vi "GraphForm (SubVI).vi"(0 "R":T1, 2 "T":T1, 5 "error in":errorcluster, 10 "Title":string) -> (19 "error out":errorcluster)   [LabVIEW 2013]
panel:
  in  "1_ch_visible":bool=TRUE
  in  "2_ch_visible":bool=TRUE
  in  "3_ch_visible":bool=TRUE
  in  "4_ch_visible":bool=TRUE
  in  "5_ch_visible":bool=TRUE
  in  "6_ch_visible":bool=TRUE
  in  "7_ch_visible":bool=TRUE
  in  "8_ch_visible":bool=TRUE
  in  "Tab Control":enum32{"Page 2"}(tab)
  in  "Autoscale":bool=TRUE
  in  "Т max":u16=300 min=2 max=500 step=1
  in  "Т min":u16=3 min=1 max=350
  in  "R max":u16=6000 min=2 max=10000 step=1
  in  "R min":u16=100 min=1 max=350
  out "часы":string="0"
  in  "Добавить время":dbl(ring)=300.0 items=["1 мин."=60.0, "5 мин."=300.0, "20 мин."=1200.0]
  out "мин.":string="1"
  in  "xScale +":bool
  in  "xScale -":bool
  out "Graphs T":dynamicdata(graph)
  out "Graphs R":dynamicdata(graph)
  # "Шкала Т"
  # "Шкала R"
  # "Интервал просмотра"
  # ":"
  # "Канал"
  # "R [Ом]"
  # "Температура, К"
  # "Сопротивление, Ом"
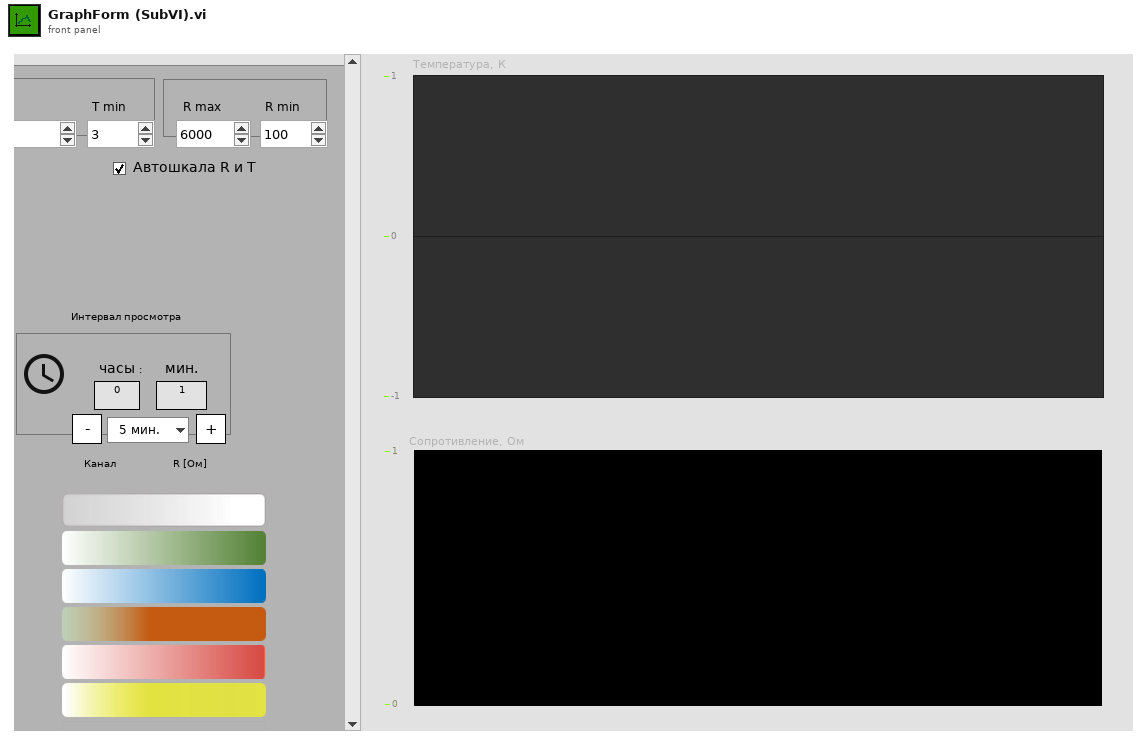
[diagram p1: front panel]
types:
  T1 = cluster{" R1":dbl, " R2":dbl, " R3":dbl, " R4":dbl, " R5":dbl, "R6":dbl, " R7":dbl, "R8":dbl}
  T2 = typedef "LVDateTimeRec.ctl" = cluster{"fractional second":dbl, "second":i32, "minute":i32, "hour":i32, "day of month":i32, "month":i32, "year":i32, "day of week":i32, "day of year":i32, "DST":i32}
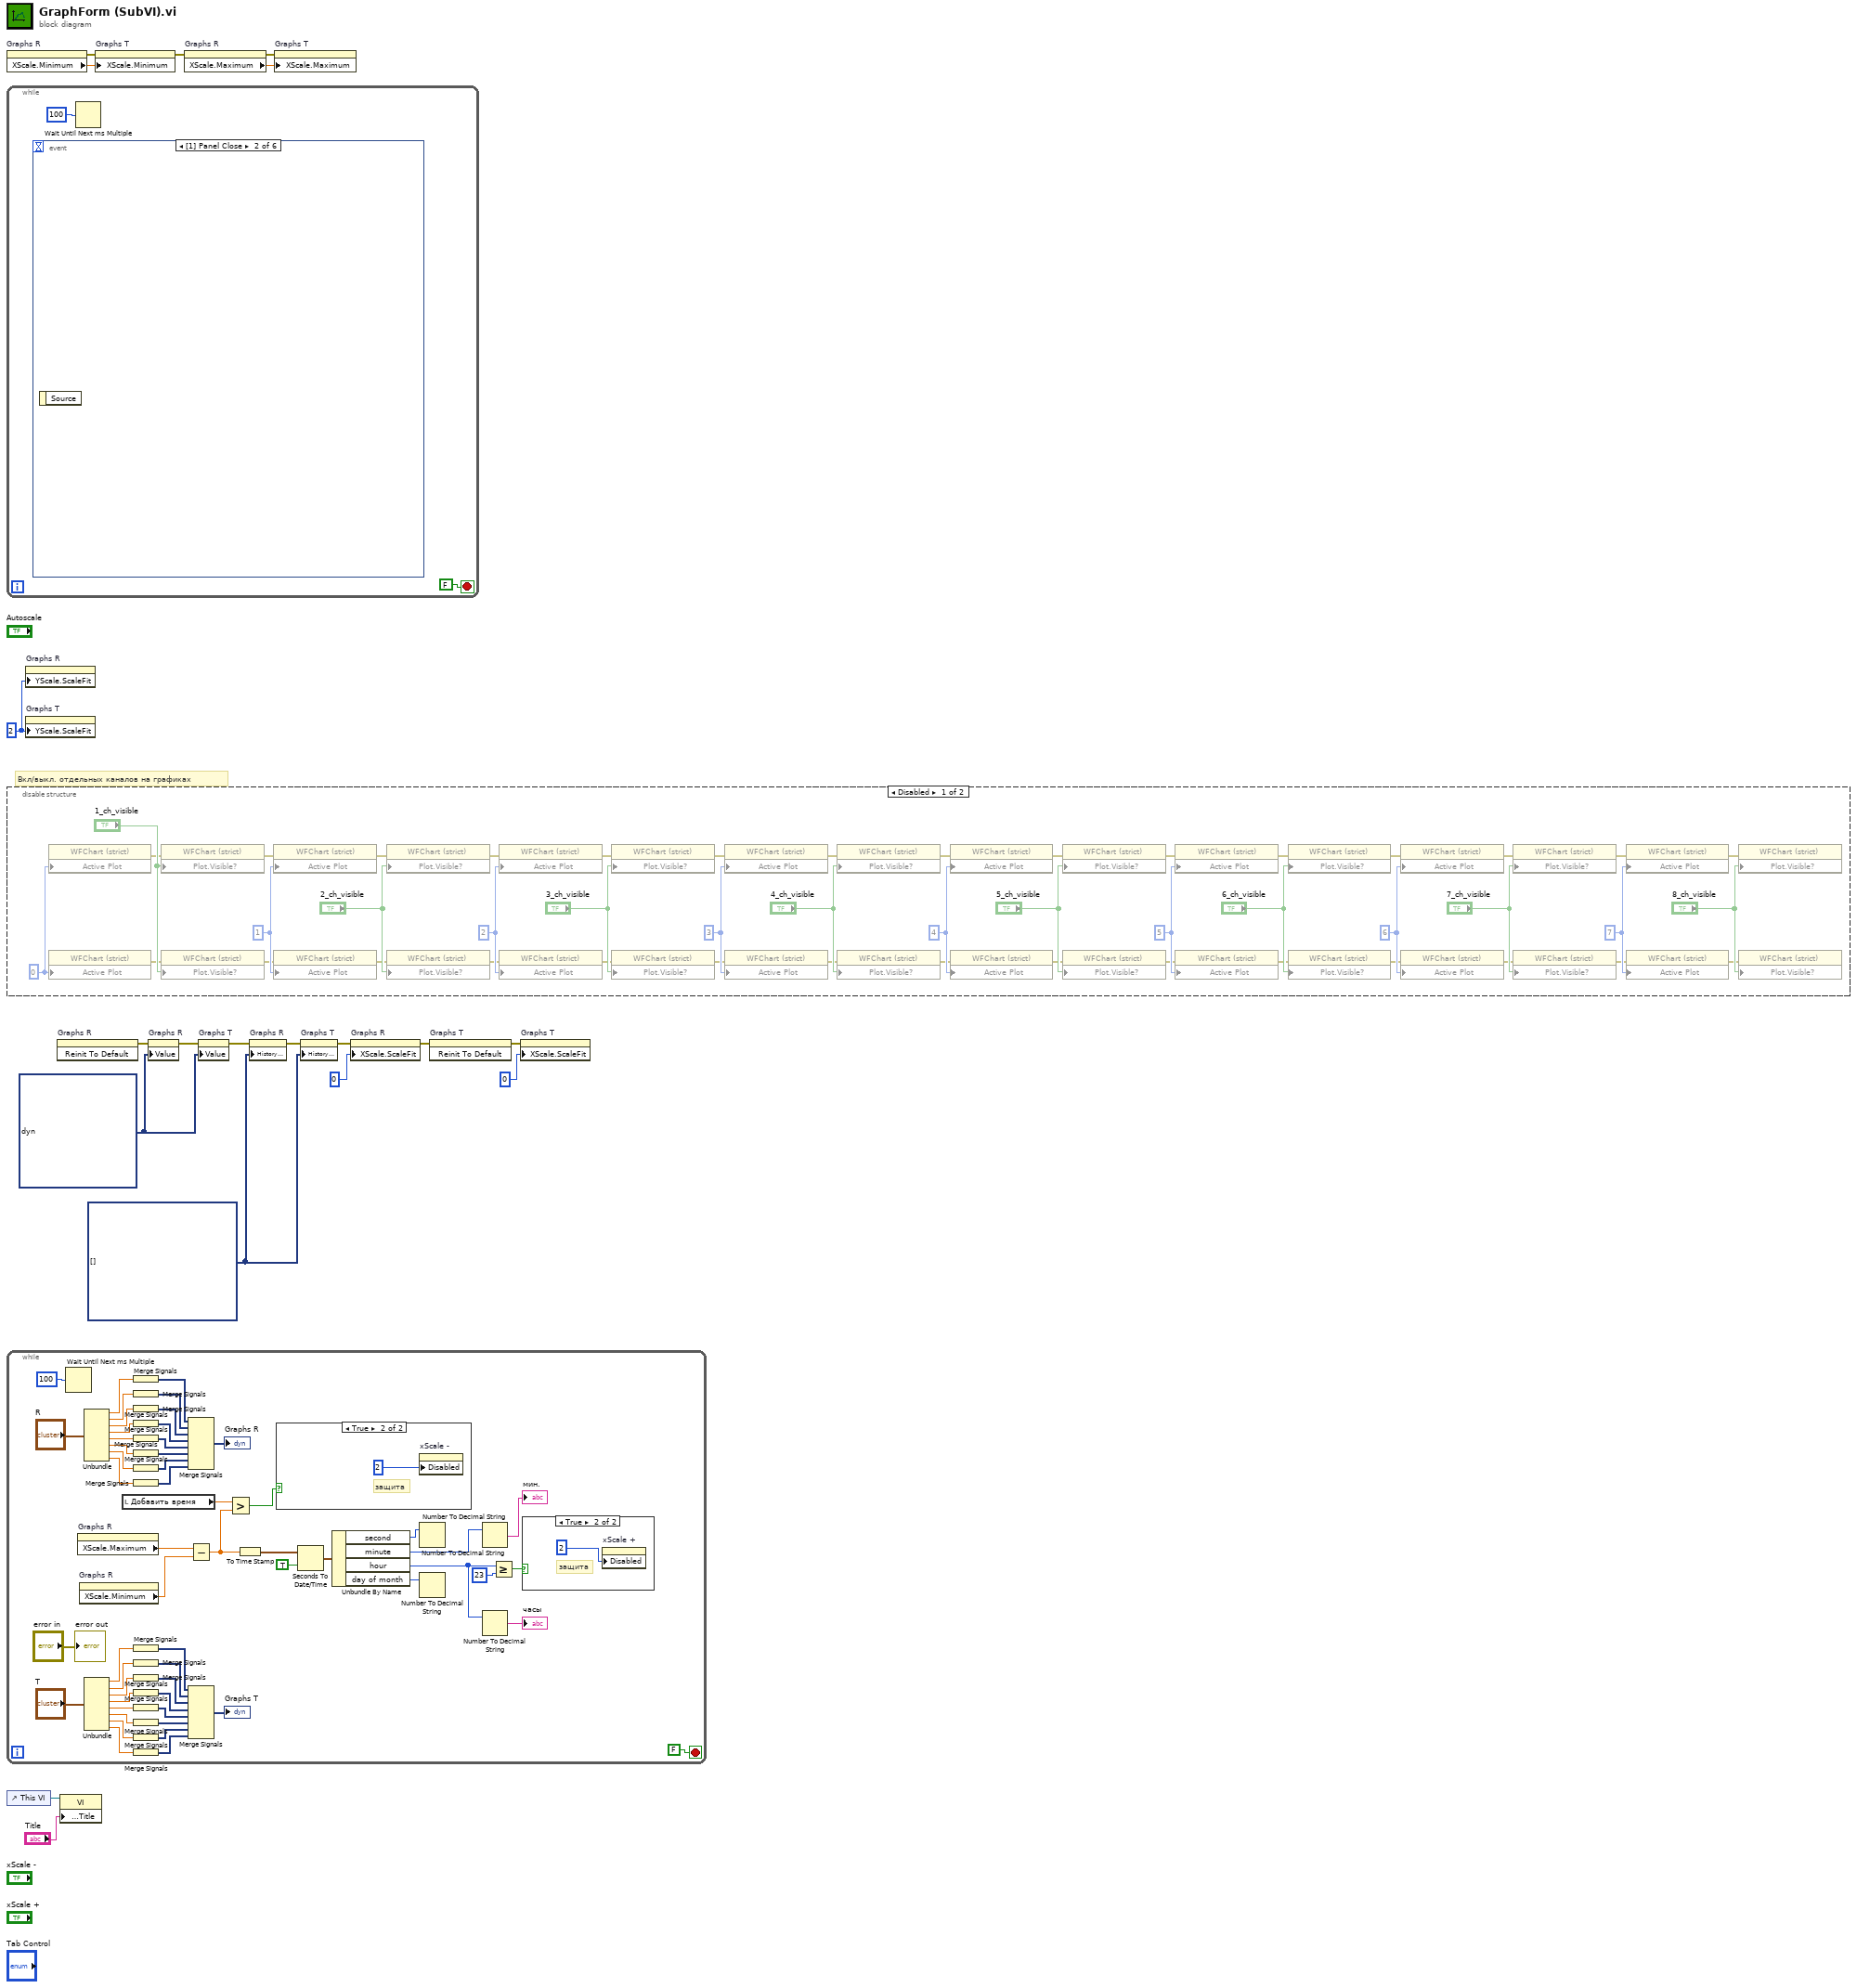
[diagram p0: block diagram]
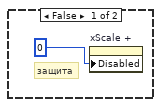
[diagram p2: hidden frame]
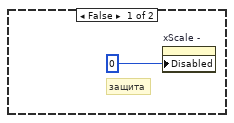
[diagram p3: hidden frame]
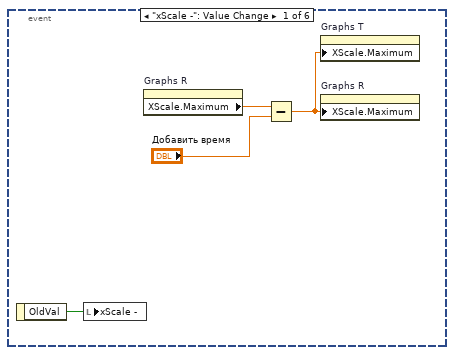
[diagram p4: hidden frame]
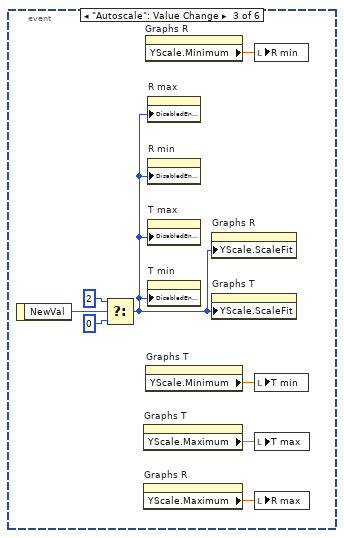
[diagram p5: hidden frame]
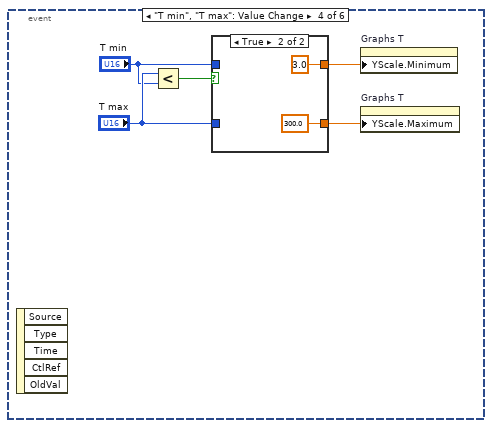
[diagram p6: hidden frame]
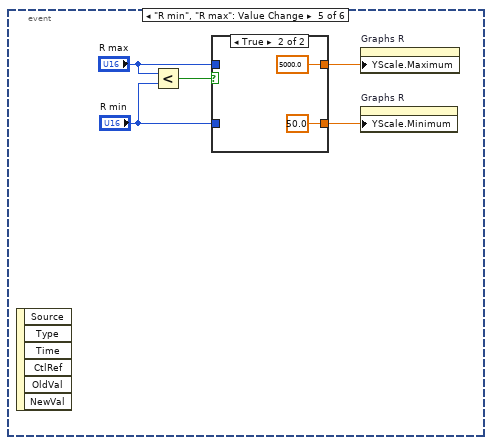
[diagram p8: hidden frame]
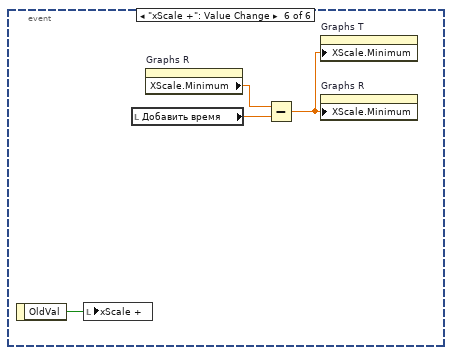
[diagram p10: hidden frame]
diagram:
  w6 = dynamicdata[] [] ("History Data")
  w7 = dynamicdata [{"t0"=timestamp(3465273261.7246556 s since 1904-01-01), "dt"=1.0, "Y"=[0.1931097262457384]}, {"t0"=timestamp(3465273261.7246556 s since 1904-01-01), "dt"=1.0, "Y"=[0.3594116459482981]}, {"t0"=timestamp(3465273261.7246556 s since 1904-01-01), "dt"=1.0, "Y"=[0.8898205452798131]}, {"t0"=timestamp(3465273261.7246556 s since 1904-01-01), "dt"=1.0, "Y"=[0.747699236883661]}] ("Graphs")
  w14 = u8 2 ("Y Scale.Scale Fit")
  # "Вкл/выкл. отдельных каналов на графиках"
  n1 = property on="Graphs R" class="WFChart (strict)"() -> (error out=w16:errorcluster, "XScale.Minimum"=w19:dbl)  [unwired: 2 in, 1 out]
  n2 = while {
    stop <- FALSE stop-if-true
    n3 = event shown="[1] Panel Close" {
      selector: _ -> [_ _ _ _ _ _]
      dyn-events: _ -> [_ _ _ _ _ _]
      timeout: _ -> [_ _ _ _ _ _]
      event "xScale -": Value Change {
        n4 = event-data() -> ("OldVal"=w25:bool)  [unwired: 1 in]
        n5 = local write "xScale -"(w25) -> ()
        n6 = property on="Graphs R" class="WFChart (strict)"() -> ("XScale.Maximum"=w23:dbl)  [unwired: 2 in, 2 out]
        n7 = Subtract(x=w23, y="Добавить время") -> (x-y=w24:dbl)
        n8 = property on="Graphs T" class="WFChart (strict)"("XScale.Maximum"=w24) -> ()  [unwired: 2 in, 2 out]
        n9 = property on="Graphs R" class="WFChart (strict)"("XScale.Maximum"=w24) -> ()  [unwired: 2 in, 2 out]
      }
      event Panel Close {
        n10 = event-data() -> ()  [unwired: 1 in, 1 out]
      }
      event "Autoscale": Value Change {
        n11 = event-data() -> ("NewVal"=w26:bool)  [unwired: 1 in]
        n12 = Select(t=u8 2 ("Y Scale.Scale Fit"), s=w26, f=u8 0 ("Y Scale.Scale Fit")) -> (s? t:f=w29:u8)
        n13 = property on="Graphs T" class="WFChart (strict)"() -> ("YScale.Maximum"=w33:dbl)  [unwired: 2 in, 2 out]
        n14 = property on="Graphs R" class="WFChart (strict)"() -> ("YScale.Maximum"=w31:dbl)  [unwired: 2 in, 2 out]
        n15 = property on="Graphs R" class="WFChart (strict)"() -> ("YScale.Minimum"=w30:dbl)  [unwired: 2 in, 2 out]
        n16 = property on="Graphs T" class="WFChart (strict)"() -> ("YScale.Minimum"=w32:dbl)  [unwired: 2 in, 2 out]
        n17 = property on="R max" class="DigNum (strict)"("DisabledEnum"=w29) -> ()  [unwired: 2 in, 2 out]
        n18 = property on="R min" class="DigNum (strict)"("DisabledEnum"=w29) -> ()  [unwired: 2 in, 2 out]
        n19 = property on="Т max" class="DigNum (strict)"("DisabledEnum"=w29) -> ()  [unwired: 2 in, 2 out]
        n20 = property on="Т min" class="DigNum (strict)"("DisabledEnum"=w29) -> ()  [unwired: 2 in, 2 out]
        n21 = property on="Graphs R" class="WFChart (strict)"("YScale.ScaleFit"=w29) -> ()  [unwired: 2 in, 2 out]
        n22 = property on="Graphs T" class="WFChart (strict)"("YScale.ScaleFit"=w29) -> ()  [unwired: 2 in, 2 out]
        n23 = local write "R min"(w30) -> ()
        n24 = local write "Т min"(w32) -> ()
        n25 = local write "Т max"(w33) -> ()
        n26 = local write "R max"(w31) -> ()
      }
      event "Т min", "Т max": Value Change {
        n27 = event-data() -> ()  [unwired: 1 in, 5 out]
        n28 = Less?(x="Т max", y="Т min") -> (x < y?=w36:bool)
        n29 = case shown="True" w36 {
          tunnel: [w39 300.0 ("x+1")] -> w38
          tunnel: [w40 3.0 ("x+1")] -> w37
          tunnel: "Т max" -> [w39 _]
          tunnel: "Т min" -> [w40 _]
          frame False {
          }
          frame True {
          }
        }
        n30 = property on="Graphs T" class="WFChart (strict)"("YScale.Minimum"=w37) -> ()  [unwired: 2 in, 2 out]
        n31 = property on="Graphs T" class="WFChart (strict)"("YScale.Maximum"=w38) -> ()  [unwired: 2 in, 2 out]
      }
      event "R min", "R max": Value Change {
        n32 = event-data() -> ()  [unwired: 1 in, 6 out]
        n33 = Less?(x="R max", y="R min") -> (x < y?=w47:bool)
        n34 = case shown="True" w47 {
          tunnel: [w48 5000.0 ("x+1")] -> w43
          tunnel: [w49 50.0 ("x+1")] -> w44
          tunnel: "R max" -> [w48 _]
          tunnel: "R min" -> [w49 _]
          frame False {
          }
          frame True {
          }
        }
        n35 = property on="Graphs R" class="WFChart (strict)"("YScale.Maximum"=w43) -> ()  [unwired: 2 in, 2 out]
        n36 = property on="Graphs R" class="WFChart (strict)"("YScale.Minimum"=w44) -> ()  [unwired: 2 in, 2 out]
      }
      event "xScale +": Value Change {
        n37 = event-data() -> ("OldVal"=w55:bool)  [unwired: 1 in]
        n38 = local write "xScale +"(w55) -> ()
        n39 = local read "Добавить время"() -> (w52:dbl)
        n40 = property on="Graphs R" class="WFChart (strict)"() -> ("XScale.Minimum"=w53:dbl)  [unwired: 2 in, 2 out]
        n41 = Subtract(x=w53, y=w52) -> (x-y=w54:dbl)
        n42 = property on="Graphs T" class="WFChart (strict)"("XScale.Minimum"=w54) -> ()  [unwired: 2 in, 2 out]
        n43 = property on="Graphs R" class="WFChart (strict)"("XScale.Minimum"=w54) -> ()  [unwired: 2 in, 2 out]
      }
    }
    n44 = Wait Until Next ms Multiple(millisecond multiple=u32 100) -> ()  [unwired: 1 out]
  }
  n45 = disable-structure shown="Disabled" {
    frame Disabled {
      w100 = u32 7 ("Active Plot")
      w98 = u32 6 ("Active Plot")
      w96 = u32 5 ("Active Plot")
      w93 = u32 4 ("Active Plot")
      w83 = u32 3 ("Active Plot")
      w80 = u32 2 ("Active Plot")
      w77 = u32 1 ("Active Plot")
      w72 = u32 0 ("Active Plot")
      n46 = property on="Property Node" class="WFChart (strict)"("Active Plot"=w72) -> (error out=w71:errorcluster)  [unwired: 2 in, 1 out]
      n47 = property on="Property Node" class="WFChart (strict)"("Active Plot"=w72) -> (error out=w59:errorcluster)  [unwired: 2 in, 1 out]
      n48 = property on="Property Node" class="WFChart (strict)"(error in=w71, "Plot.Visible?"="1_ch_visible") -> (error out=w78:errorcluster)  [unwired: 1 in, 1 out]
      n49 = property on="Property Node" class="WFChart (strict)"(error in=w59, "Plot.Visible?"="1_ch_visible") -> (error out=w57:errorcluster)  [unwired: 1 in, 1 out]
      n50 = property on="Property Node" class="WFChart (strict)"(error in=w78, "Active Plot"=w77) -> (error out=w74:errorcluster)  [unwired: 1 in, 1 out]
      n51 = property on="Property Node" class="WFChart (strict)"(error in=w57, "Active Plot"=w77) -> (error out=w58:errorcluster)  [unwired: 1 in, 1 out]
      n52 = property on="Property Node" class="WFChart (strict)"(error in=w74, "Plot.Visible?"="2_ch_visible") -> (error out=w81:errorcluster)  [unwired: 1 in, 1 out]
      n53 = property on="Property Node" class="WFChart (strict)"(error in=w58, "Plot.Visible?"="2_ch_visible") -> (error out=w56:errorcluster)  [unwired: 1 in, 1 out]
      n54 = property on="Property Node" class="WFChart (strict)"(error in=w81, "Active Plot"=w80) -> (error out=w75:errorcluster)  [unwired: 1 in, 1 out]
      n55 = property on="Property Node" class="WFChart (strict)"(error in=w56, "Active Plot"=w80) -> (error out=w70:errorcluster)  [unwired: 1 in, 1 out]
      n56 = property on="Property Node" class="WFChart (strict)"(error in=w75, "Plot.Visible?"="3_ch_visible") -> (error out=w84:errorcluster)  [unwired: 1 in, 1 out]
      n57 = property on="Property Node" class="WFChart (strict)"(error in=w70, "Plot.Visible?"="3_ch_visible") -> (error out=w69:errorcluster)  [unwired: 1 in, 1 out]
      n58 = property on="Property Node" class="WFChart (strict)"(error in=w84, "Active Plot"=w83) -> (error out=w76:errorcluster)  [unwired: 1 in, 1 out]
      n59 = property on="Property Node" class="WFChart (strict)"(error in=w69, "Active Plot"=w83) -> (error out=w68:errorcluster)  [unwired: 1 in, 1 out]
      n60 = property on="Property Node" class="WFChart (strict)"(error in=w76, "Plot.Visible?"="4_ch_visible") -> (error out=w94:errorcluster)  [unwired: 1 in, 1 out]
      n61 = property on="Property Node" class="WFChart (strict)"(error in=w68, "Plot.Visible?"="4_ch_visible") -> (error out=w60:errorcluster)  [unwired: 1 in, 1 out]
      n62 = property on="Property Node" class="WFChart (strict)"(error in=w94, "Active Plot"=w93) -> (error out=w92:errorcluster)  [unwired: 1 in, 1 out]
      n63 = property on="Property Node" class="WFChart (strict)"(error in=w60, "Active Plot"=w93) -> (error out=w61:errorcluster)  [unwired: 1 in, 1 out]
      n64 = property on="Property Node" class="WFChart (strict)"(error in=w92, "Plot.Visible?"="5_ch_visible") -> (error out=w88:errorcluster)  [unwired: 1 in, 1 out]
      n65 = property on="Property Node" class="WFChart (strict)"(error in=w61, "Plot.Visible?"="5_ch_visible") -> (error out=w63:errorcluster)  [unwired: 1 in, 1 out]
      n66 = property on="Property Node" class="WFChart (strict)"(error in=w88, "Active Plot"=w96) -> (error out=w91:errorcluster)  [unwired: 1 in, 1 out]
      n67 = property on="Property Node" class="WFChart (strict)"(error in=w63, "Active Plot"=w96) -> (error out=w62:errorcluster)  [unwired: 1 in, 1 out]
      n68 = property on="Property Node" class="WFChart (strict)"(error in=w91, "Plot.Visible?"="6_ch_visible") -> (error out=w87:errorcluster)  [unwired: 1 in, 1 out]
      n69 = property on="Property Node" class="WFChart (strict)"(error in=w62, "Plot.Visible?"="6_ch_visible") -> (error out=w65:errorcluster)  [unwired: 1 in, 1 out]
      n70 = property on="Property Node" class="WFChart (strict)"(error in=w87, "Active Plot"=w98) -> (error out=w90:errorcluster)  [unwired: 1 in, 1 out]
      n71 = property on="Property Node" class="WFChart (strict)"(error in=w65, "Active Plot"=w98) -> (error out=w64:errorcluster)  [unwired: 1 in, 1 out]
      n72 = property on="Property Node" class="WFChart (strict)"(error in=w90, "Plot.Visible?"="7_ch_visible") -> (error out=w86:errorcluster)  [unwired: 1 in, 1 out]
      n73 = property on="Property Node" class="WFChart (strict)"(error in=w64, "Plot.Visible?"="7_ch_visible") -> (error out=w67:errorcluster)  [unwired: 1 in, 1 out]
      n74 = property on="Property Node" class="WFChart (strict)"(error in=w86, "Active Plot"=w100) -> (error out=w89:errorcluster)  [unwired: 1 in, 1 out]
      n75 = property on="Property Node" class="WFChart (strict)"(error in=w67, "Active Plot"=w100) -> (error out=w66:errorcluster)  [unwired: 1 in, 1 out]
      n76 = property on="Property Node" class="WFChart (strict)"(error in=w89, "Plot.Visible?"="8_ch_visible") -> ()  [unwired: 1 in, 2 out]
      n77 = property on="Property Node" class="WFChart (strict)"(error in=w66, "Plot.Visible?"="8_ch_visible") -> ()  [unwired: 1 in, 2 out]
    }
    frame Enabled {
    }
  }
  n78 = while {
    stop <- FALSE stop-if-true
    n79 = Wait Until Next ms Multiple(millisecond multiple=u32 100) -> ()  [unwired: 1 out]
    n80 = property on="Graphs R" class="WFChart (strict)"() -> ("XScale.Maximum"=w156:dbl)  [unwired: 2 in, 2 out]
    n81 = property on="Graphs R" class="WFChart (strict)"() -> ("XScale.Minimum"=w155:dbl)  [unwired: 2 in, 2 out]
    n82 = Unbundle("R") -> ("R1"=w130:dbl, "R2"=w129:dbl, "R3"=w128:dbl, "R4"=w127:dbl, "R5"=w126:dbl, "R6"=w125:dbl, "R7"=w124:dbl, "R8"=w123:dbl)
    n83 = Unbundle("T") -> ("R1"=w115:dbl, "R2"=w116:dbl, "R3"=w117:dbl, "R4"=w118:dbl, "R5"=w119:dbl, "R6"=w120:dbl, "R7"=w121:dbl, "R8"=w122:dbl)
    n84 = local read "Добавить время"() -> (w153:dbl)
    n85 = Merge Signals(w130) -> (w137:dynamicdata)
    n86 = Merge Signals(w129) -> (w136:dynamicdata)
    n87 = Merge Signals(w128) -> (w135:dynamicdata)
    n88 = Merge Signals(w127) -> (w138:dynamicdata)
    n89 = Merge Signals(w126) -> (w133:dynamicdata)
    n90 = Merge Signals(w125) -> (w132:dynamicdata)
    n91 = Merge Signals(w124) -> (w131:dynamicdata)
    n92 = Merge Signals(w123) -> (w134:dynamicdata)
    n93 = Merge Signals(w115) -> (w108:dynamicdata)
    n94 = Merge Signals(w116) -> (w109:dynamicdata)
    n95 = Merge Signals(w117) -> (w110:dynamicdata)
    n96 = Merge Signals(w118) -> (w107:dynamicdata)
    n97 = Merge Signals(w119) -> (w112:dynamicdata)
    n98 = Merge Signals(w120) -> (w113:dynamicdata)
    n99 = Merge Signals(w121) -> (w114:dynamicdata)
    n100 = Merge Signals(w122) -> (w111:dynamicdata)
    n101 = Merge Signals(w137, w136, w135, w138, w133, w132, w131, w134) -> (→"Graphs R":dynamicdata)
    n102 = Subtract(x=w156, y=w155) -> (x-y=w146:dbl)
    n103 = Merge Signals(w108, w109, w110, w107, w112, w113, w114, w111) -> (→"Graphs T":dynamicdata)
    n104 = Greater?(x=w153, y=w146) -> (0:w154:bool)
    n105 = To Time Stamp(1:w146) -> (0:w151:timestamp)
    n106 = case shown="True" w154 {
      frame False {
        # "защита"
        n107 = property on="xScale -" class="Bool (strict)"("Disabled"=u8 0) -> ()  [unwired: 2 in, 2 out]
      }
      frame True {
        # "защита"
        n108 = property on="xScale -" class="Bool (strict)"("Disabled"=u8 2) -> ()  [unwired: 2 in, 2 out]
      }
    }
    n109 = Seconds To Date/Time(time stamp (now)=w151, to UTC (F)=TRUE) -> (date time rec=w150:T2)
    n110 = Unbundle By Name(w150) -> ("second"=w149:i32, "minute"=w148:i32, "hour"=w144:i32, "day of month"=w147:i32)
    n111 = Number To Decimal String(number=w149) -> ()  [unwired: 2 out]
    n112 = Number To Decimal String(number=w147) -> ()  [unwired: 2 out]
    n113 = Number To Decimal String(number=w148) -> (decimal integer string=→"мин.":string)  [unwired: 1 out]
    n114 = Number To Decimal String(number=w144) -> (decimal integer string=→"часы":string)  [unwired: 1 out]
    n115 = Greater Or Equal?(x=w144, y=23) -> (x >= y?=w145:bool)
    n116 = case shown="True" w145 {
      frame False {
        # "защита"
        n117 = property on="xScale +" class="Bool (strict)"("Disabled"=u8 0) -> ()  [unwired: 2 in, 2 out]
      }
      frame True {
        # "защита"
        n118 = property on="xScale +" class="Bool (strict)"("Disabled"=u8 2) -> ()  [unwired: 2 in, 2 out]
      }
    }
    "error out" <- "error in"
  }
  n119 = control-ref of="This VI"() -> (w13:refnum<vi>)
  n120 = property on="Graphs R" class="WFChart (strict)"("YScale.ScaleFit"=w14) -> ()  [unwired: 2 in, 2 out]
  n121 = property on="Graphs T" class="WFChart (strict)"("YScale.ScaleFit"=w14) -> ()  [unwired: 2 in, 2 out]
  n122 = invoke on="Graphs R" class="WFChart (strict)" method="Reinit To Default"() -> (error out=w11:errorcluster)  [unwired: 3 in, 2 out]
  n123 = property class="VI"(reference=w13, "Front Panel.Title"="Title") -> ()  [unwired: 1 in, 2 out]
  n124 = property on="Graphs T" class="WFChart (strict)"(error in=w16, "XScale.Minimum"=w19) -> (error out=w17:errorcluster)  [unwired: 1 in, 1 out]
  n125 = property on="Graphs R" class="WFChart (strict)"(error in=w11, "Value"=w7) -> (error out=w5:errorcluster)  [unwired: 1 in, 1 out]
  n126 = property on="Graphs R" class="WFChart (strict)"(error in=w17) -> (error out=w15:errorcluster, "XScale.Maximum"=w18:dbl)  [unwired: 1 in, 1 out]
  n127 = property on="Graphs T" class="WFChart (strict)"(error in=w5, "Value"=w7) -> (error out=w4:errorcluster)  [unwired: 1 in, 1 out]
  n128 = property on="Graphs R" class="WFChart (strict)"(error in=w4, "History Data"=w6) -> (error out=w3:errorcluster)  [unwired: 1 in, 1 out]
  n129 = property on="Graphs T" class="WFChart (strict)"(error in=w15, "XScale.Maximum"=w18) -> ()  [unwired: 1 in, 2 out]
  n130 = property on="Graphs T" class="WFChart (strict)"(error in=w3, "History Data"=w6) -> (error out=w2:errorcluster)  [unwired: 1 in, 1 out]
  n131 = property on="Graphs R" class="WFChart (strict)"(error in=w2, "XScale.ScaleFit"=u8 0 ("Y Scale.Scale Fit")) -> (error out=w9:errorcluster)  [unwired: 1 in, 1 out]
  n132 = invoke on="Graphs T" class="WFChart (strict)" method="Reinit To Default"(error in=w9) -> (error out=w1:errorcluster)  [unwired: 2 in, 2 out]
  n133 = property on="Graphs T" class="WFChart (strict)"(error in=w1, "XScale.ScaleFit"=u8 0 ("Y Scale.Scale Fit")) -> ()  [unwired: 1 in, 2 out]
